vi "DCS_Signal_Amp_peak.vi"(10 "data":waveform(dbl)[](array[waveform])) -> (0 "Data":dbl[](array[numeric]))   [LabVIEW 2012]
panel:
  out "Filtered Signal":waveform(dbl)[](graph)
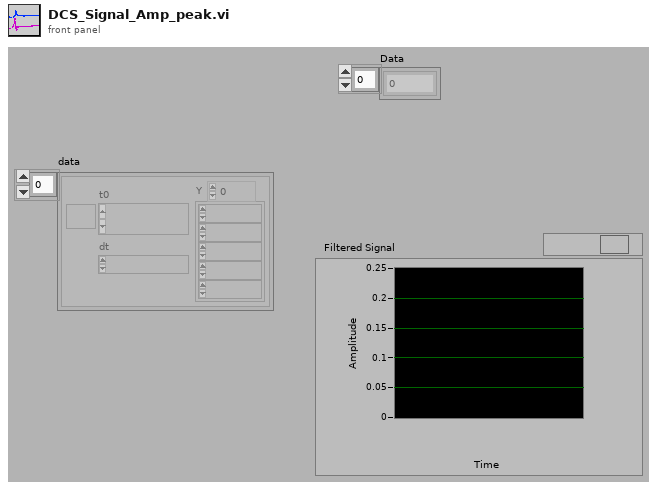
[diagram p1: front panel]
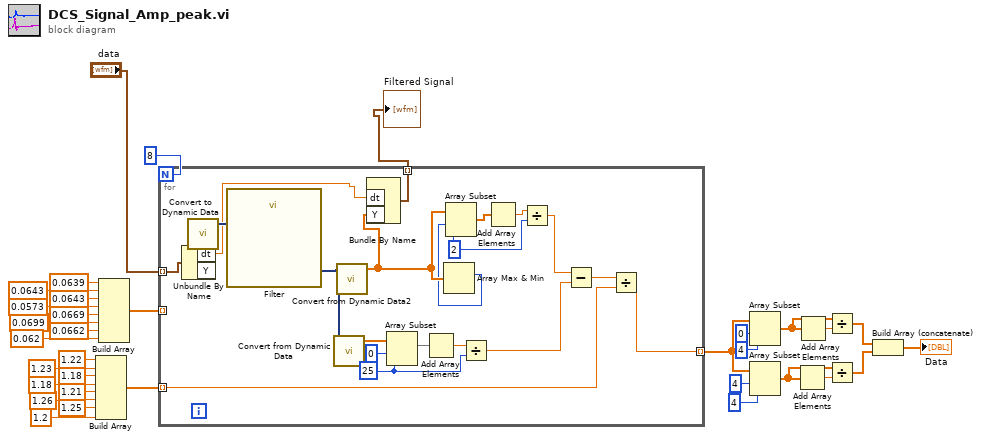
[diagram p0: block diagram]
diagram:
  n1 = Build Array(1.22 ("element"), 1.23 ("element"), 1.18 ("element"), 1.18 ("element"), 1.21 ("element"), 1.26 ("element"), 1.25 ("element"), 1.2 ("element")) -> (w14:dbl[])
  n2 = Build Array(0.0639 ("element"), 0.0643 ("element"), 0.0643 ("element"), 0.0573 ("element"), 0.0669 ("element"), 0.0699 ("element"), 0.0662 ("element"), 0.062 ("element")) -> (w23:dbl[])
  n3 = for {
    N: 8 -> [_]
    tunnel: "data" -> [w38] mode=indexing
    tunnel: w23 -> [_] mode=indexing
    tunnel: w14 -> [w53] mode=indexing
    tunnel: [w52] -> w10 mode=indexing
    tunnel: [w37] -> w1 mode=indexing
    w41 = 2 ("length")
    w48 = 25 ("length")
    n4 = Unbundle By Name(w38) -> ("dt"=w34:dbl, "Y"=w46:dbl[])
    n5 = call "Convert to Dynamic Data"("Array"=w46) -> ("Dynamic Data Type"=w45:dynamicdata)  [unwired: 3 in]
    n6 = call "Filter"("Signal"=w45) -> ("Filtered Signal"=w39:dynamicdata)  [unwired: 9 in, 1 out]
    n7 = call "Convert from Dynamic Data"("Dynamic Data Type"=w39) -> ("Array"=w44:dbl[])  [unwired: 3 in]
    n8 = call "Convert from Dynamic Data2"("Dynamic Data Type"=w39) -> ("Array"=w36:dbl[])  [unwired: 3 in]
    n9 = Bundle By Name("dt"=w34, "Y"=w36) -> (w37:waveform(dbl))  [unwired: 1 in]
    n10 = Array Subset(array=w44, index=0, length=w48) -> (w51:dbl[])
    n11 = Add Array Elements(numeric array=w51) -> (sum=w49:dbl)
    n12 = Array Max & Min(array=w36) -> (max index (indices)=w35:i32)  [unwired: 3 out]
    n13 = Array Subset(array=w36, index=w35, length=w41) -> (w43:dbl[])
    n14 = Divide(x=w49, y=w48) -> (x/y=w47:dbl)
    n15 = Add Array Elements(numeric array=w43) -> (sum=w42:dbl)
    n16 = Divide(x=w42, y=w41) -> (x/y=w40:dbl)
    n17 = Subtract(x=w40, y=w47) -> (x-y=w54:dbl)
    n18 = Divide(x=w54, y=w53) -> (x/y=w52:dbl)
  }
  "Filtered Signal" <- w1
  n19 = Array Subset(array=w10, index=0, length=4) -> (w6:dbl[])
  n20 = Array Subset(array=w10, index=4, length=4) -> (w7:dbl[])
  n21 = Add Array Elements(numeric array=w7) -> (sum=w8:dbl)
  n22 = Add Array Elements(numeric array=w6) -> (sum=w9:dbl)
  n23 = Divide(x=w6, y=w9) -> (x/y=w5:dbl[])
  n24 = Divide(x=w7, y=w8) -> (x/y=w4:dbl[])
  n25 = Build Array (concatenate)(w5, w4) -> (→"Data":dbl[])
